vi "Find Circle VI.vi"(0 "Image In":T6, 1 "Image Dst":T6, 2 "ROI Descriptor (Find Circular Edge 1)":T5={"Global Rectangle"=[157, 187, 247, 277], "Contours"=[{"ID"=enum."External", "Type"=7, "Coordinates"=[201, 231, 20, 44, 0, 264958]}]} {"Contours"."Type" items=["No Selection", "Point", "Line", "Rectangle", "Oval", "Polygon", "Freehand Region", "Annulus", "Unused2", "Unused3", "Broken Line", "Freehand Line", "Rotated Rectangle"]}, 3 "Options (Find Circular Edge 1)":T4={"Search  Direction"=0, "Edge Options"={"Edge Polarity"=0, "Kernel Size"=3, "Width"=5, "Minimum Edge Strength"=50.0, "Interpolation Type"=enum."Bilinear Fixed", "Data Processing Method"=enum."Average"}, "Show Search Area"=TRUE, "Show Search Lines"=TRUE, "Show Edges Found"=TRUE, "Show Result"=TRUE, "Search Area Color"=65280, "Search Lines Color"=255, "Edge Locations Color"=16776960, "Result Color"=16711680, "Overlay Group Name"=""} {"Search  Direction" items=["Outside to Inside", "Inside to Outside"]; "Edge Options"."Edge Polarity" items=["All Edges", "Rising Edges", "Falling Edges"]; "Edge Options"."Minimum Edge Strength" format="%.2f"; "Edge Options"."Width" step=2; "Edge Options"."Kernel Size" step=2}, 4 "Circle Fit Options (Find Circular Edge 1)":T1={"Process"=enum."Get Best Edge", "Step Size"=14, "Max Pixel Radius"=3}, 7 "error in":errorcluster) -> (20 "Image Out":T6, 21 "Fitted Circle (Find Circular Edge 1)":T7 {"Average SNR (dB)" format="%.2f"; "Average Strength" format="%.2f"; "Roundness (Real-World)" format="%.2f"; "Radius (Real-World)" format="%.2f"; "Center (Real-World)"."Y" format="%.2f"; "Center (Real-World)"."X" format="%.2f"; "Radius (Pixels)" format="%.2f"; "Center (Pixels)"."Y" format="%.2f"; "Center (Pixels)"."X" format="%.2f"}, 27 "error out":errorcluster)   [LabVIEW 2020]
doc: "Creates, edits, and runs vision algorithms using NI Vision Assistant.\n\nWhen you place this Express VI on the block diagram, NI Vision Assistant launches. Create an algorithm using the Vision Assistant processing functions. After you create an algorithm, you can select the controls and indicators that you want to be able to programmatically set in LabVIEW. Double-click the Vision Assistant Express VI to edit the algorithm."
uses:
  <vilib>/vision/Image Controls.llb/IMAQ Image.ctl
  <vilib>/vision/Measure.llb/Edge Options.ctl
  <vilib>/vision/Measure.llb/Edge Polarity.ctl
  <vilib>/vision/NI_Vision_Development_Module.lvlib
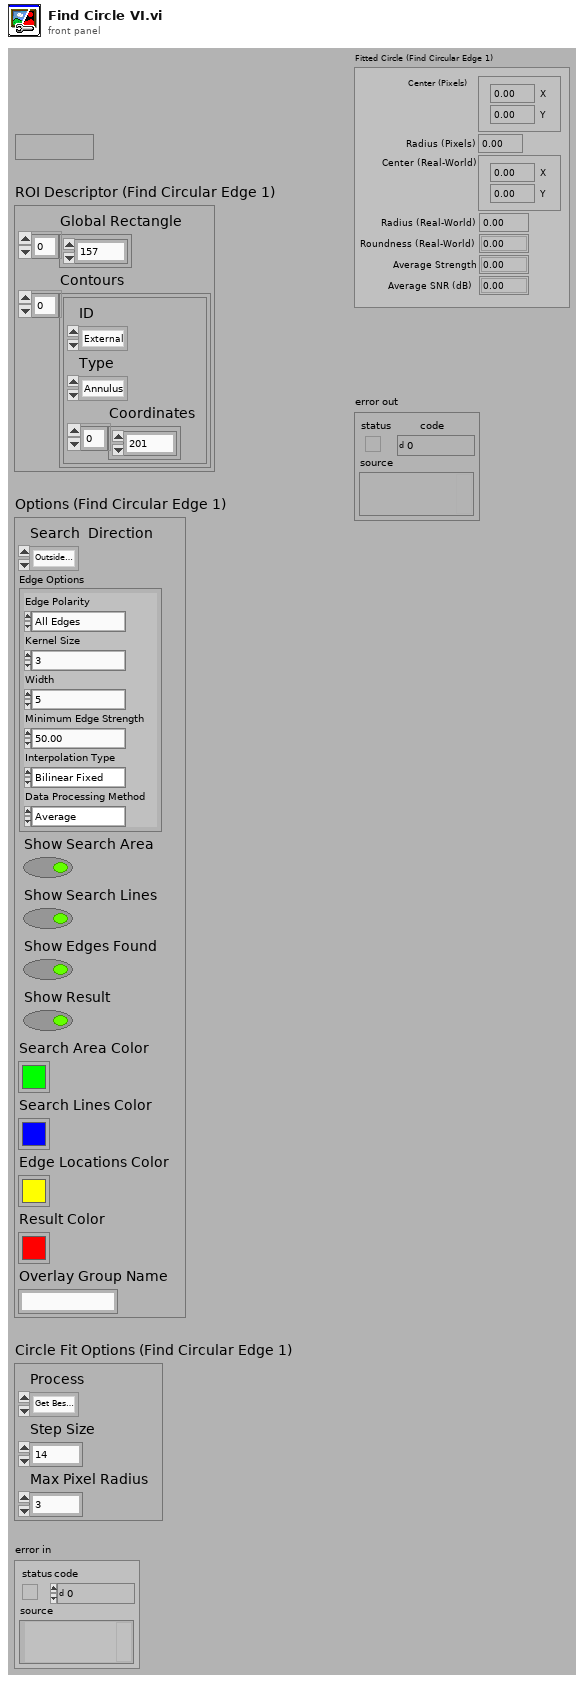
[diagram p1: front panel]
types:
  T1 = cluster{"Process":enum16{"Get First Edge", "Get First + Last Edge", "Get All Edges", "Get Best Edge"}, "Step Size":i32, "Max Pixel Radius":i32}
  T2 = typedef "Edge Options.ctl" = cluster{"Edge Polarity":T3, "Kernel Size":u32, "Width":u32, "Minimum Edge Strength":sgl, "Interpolation Type":enum32{"Zero Order", "Bilinear", "Quadratic", "Cubic", "Bilinear Fixed"}, "Data Processing Method":enum32{"Average", "Median"}}
  T3 = typedef "Edge Polarity.ctl" = u32
  T4 = cluster{"Search  Direction":u32, "Edge Options":T2, "Show Search Area":bool, "Show Search Lines":bool, "Show Edges Found":bool, "Show Result":bool, "Search Area Color":u32, "Search Lines Color":u32, "Edge Locations Color":u32, "Result Color":u32, "Overlay Group Name":string}
  T5 = cluster{"Global Rectangle":i32[], "Contours":cluster{"ID":enum32{"External", "Internal"}, "Type":u32, "Coordinates":i32[]}[]}
  T6 = typedef "IMAQ Image.ctl" = refnum<image>
  T7 = cluster{"Center (Pixels)":cluster{"X":sgl, "Y":sgl}, "Radius (Pixels)":dbl, "Center (Real-World)":cluster{"X":sgl, "Y":sgl}, "Radius (Real-World)":dbl, "Roundness (Real-World)":dbl, "Average Strength":dbl, "Average SNR (dB)":dbl}
  T8 = typedef "Image Type" = u32
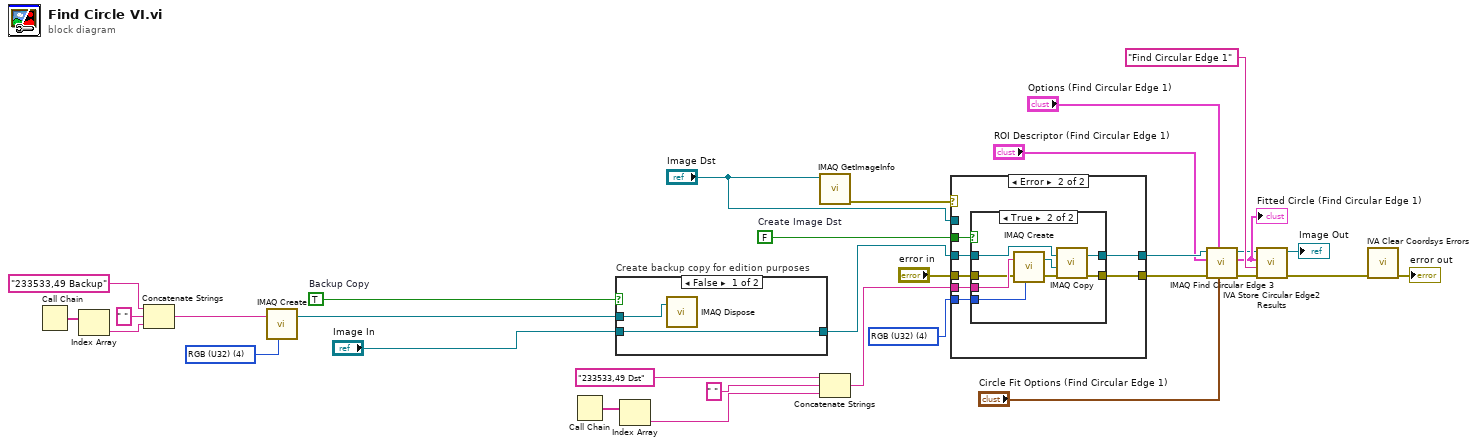
[diagram p0: block diagram]
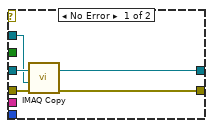
[diagram p2: hidden frame]
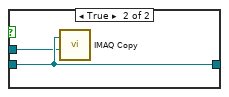
[diagram p4: hidden frame]
diagram:
  w13 = T8 4 items=["Grayscale (U8)", "Grayscale (I16)", "Grayscale (SGL)", "Complex (CSG)", "RGB (U32)", "HSL (U32)", "RGB (U64)", "Grayscale (U16)"] ("Image Dst Type")
  w14 = T8 4 items=["Grayscale (U8)", "Grayscale (I16)", "Grayscale (SGL)", "Complex (CSG)", "RGB (U32)", "HSL (U32)", "RGB (U64)", "Grayscale (U16)"] ("Image Type")
  w32 = TRUE  # Backup Copy
  w26 = FALSE  # Create Image Dst
  n1 = Call Chain() -> (call chain=w20:string[])
  n2 = Index Array(array=w20) -> (element=w19:string)  [unwired: 1 in]
  n3 = Concatenate Strings("233533,49 Backup" ("Backup Image Name"), " ", w19) -> (w16:string)
  n4 = call "IMAQ Create"("Image Name"=w16, "Image Type"=w14) -> ("New Image"=w15:T6)  [unwired: 2 in, 2 out]
  n5 = Call Chain() -> (call chain=w25:string[])
  n6 = case "Create backup copy for edition purposes" shown="False" w32 {
    tunnel: [w34 w36] -> w28
    tunnel: "Image In" -> [w34 w36]
    tunnel: w15 -> [w33 w35]
    frame False {
      n7 = call "IMAQ Dispose"("Image"=w33) -> ()  [unwired: 2 in, 4 out]
    }
    frame True {
      n8 = call "IMAQ Copy"("Image Dst"=w35, "Image Src"=w36) -> ()  [unwired: 1 in, 5 out]
    }
  }
  n9 = Index Array(array=w25) -> (element=w23:string)  [unwired: 1 in]
  n10 = call "IMAQ GetImageInfo"("Image"="Image Dst") -> ("error out"=w30:errorcluster)  [unwired: 1 in, 9 out]
  n11 = Concatenate Strings("233533,49 Dst" ("Image Dst Name"), " ", w23) -> (w21:string)
  n12 = case shown="Error" w30 {
    tunnel: [w41 w45] -> w12
    tunnel: [w40 w44] -> w9
    tunnel: w28 -> [w39 w46]
    tunnel: "error in" -> [w38 w42]
    tunnel: "Image Dst" -> [w37 _]
    tunnel: w21 -> [_ w48]
    tunnel: w13 -> [_ w47]
    tunnel: w26 -> [_ w43]
    frame No Error {
      n13 = call "IMAQ Copy"("error in (no error)"=w38, "Image Dst"=w37, "Image Src"=w39) -> ("error out"=w40:errorcluster, "Image Dst Out"=w41:T6)  [unwired: 3 out]
    }
    frame Error {
      n14 = case shown="True" w43 {
        tunnel: w48 -> [_ w58]
        tunnel: w47 -> [_ w57]
        tunnel: w46 -> [w50 w55]
        tunnel: [w50 w54] -> w45
        tunnel: [w49 w53] -> w44
        tunnel: w42 -> [w49 w51]
        frame False {
        }
        frame True {
          n15 = call "IMAQ Create"("Image Name"=w58, "Image Type"=w57, "error in (no error)"=w51) -> ("New Image"=w56:T6, "error out"=w52:errorcluster)  [unwired: 1 in, 1 out]
          n16 = call "IMAQ Copy"("error in (no error)"=w52, "Image Dst"=w56, "Image Src"=w55) -> ("error out"=w53:errorcluster, "Image Dst Out"=w54:T6)  [unwired: 3 out]
        }
      }
    }
  }
  n17 = call "IMAQ Find Circular Edge 3"("Circle Fit Options"="Circle Fit Options (Find Circular Edge 1)", "Options"="Options (Find Circular Edge 1)", "error in (no error)"=w9, "ROI Descriptor"="ROI Descriptor (Find Circular Edge 1)", "Image"=w12) -> ("error out"=w5:errorcluster, "Fitted Circle"=w7:T7, "Image Out"=w4:T6)  [unwired: 2 in, 2 out]
  "Fitted Circle (Find Circular Edge 1)" <- w7
  n18 = call <vilib>:"IVA Store Circular Edge2 Results.vi"("error in (no error)"=w5, "Step Name"="Find Circular Edge 1", "Fitted Circle"=w7, "Image in"=w4) -> ("error out"=w3:errorcluster, "Image dup"=→"Image Out":T6)  [unwired: 2 in, 4 out]
  n19 = call <vilib>:"IVA Clear Coordsys Errors.vi"("error in (no error)"=w3) -> ("error out"=→"error out":errorcluster)  [unwired: 10 in]
